vi "Escribir.vi"(2 "error out":errorcluster, 3 "VISA resource name out":refnum<visa-resource-name>, 4 "Servo ON":bool, 5 "System ON":bool) -> (0 "error out 2":errorcluster, 1 "VISA resource name out 2":refnum<visa-resource-name>)   [LabVIEW 2015, in "Arduino GIERM.lvlib"]
uses:
  <instrlib>/Arduino GIERM/Arduino GIERM.lvlib
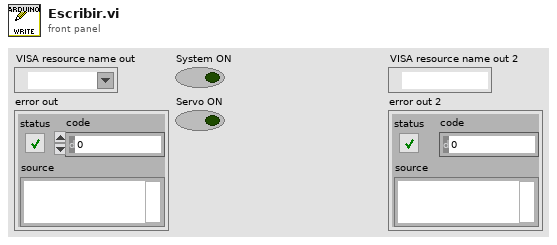
[diagram p1: front panel]
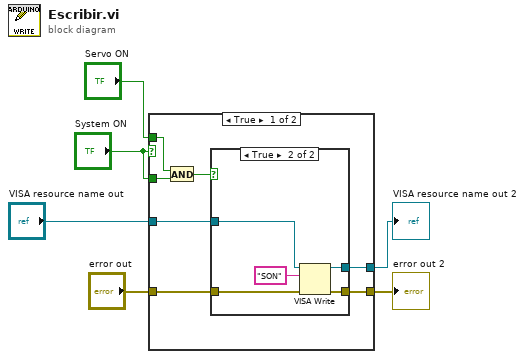
[diagram p0: block diagram]
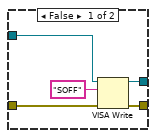
[diagram p2: hidden frame]
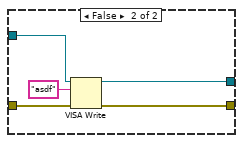
[diagram p3: hidden frame]
diagram:
  n1 = case shown="True" "System ON" {
    tunnel: [w11 w28] -> w2
    tunnel: [w10 w27] -> w1
    tunnel: "VISA resource name out" -> [w13 w26]
    tunnel: "error out" -> [w12 w25]
    tunnel: "System ON" -> [w9 _]
    tunnel: "Servo ON" -> [w8 _]
    frame True {
      n2 = And(x=w8, y=w9) -> (x .and. y?=w7:bool)
      n3 = case shown="True" w7 {
        tunnel: w13 -> [w15 w23]
        tunnel: w12 -> [w14 w22]
        tunnel: [w16 w21] -> w10
        tunnel: [w17 w20] -> w11
        frame False {
          n4 = VISA Write(VISA resource name=w15, write buffer="SOFF", error in (no error)=w14) -> (VISA resource name out=w17:refnum<visa-resource-name>, error out=w16:errorcluster)  [unwired: 1 out]
        }
        frame True {
          n5 = VISA Write(VISA resource name=w23, write buffer="SON", error in (no error)=w22) -> (VISA resource name out=w20:refnum<visa-resource-name>, error out=w21:errorcluster)  [unwired: 1 out]
        }
      }
    }
    frame False {
      n6 = VISA Write(VISA resource name=w26, write buffer="asdf", error in (no error)=w25) -> (VISA resource name out=w28:refnum<visa-resource-name>, error out=w27:errorcluster)  [unwired: 1 out]
    }
  }
  "VISA resource name out 2" <- w2
  "error out 2" <- w1
